vi "LED_Load_Ref-Offset.vi"(0 "Load Resource in":refnum<k15>, 1 "Max Output Resistance":string, 2 "Cluster":T1, 5 "Aperture time":dbl, 7 "Load channel name":string, 9 "DUT Current Limit":dbl, 11 "error in":errorcluster, 12 "Load voltage limit range":dbl) -> (4 "Load Resource Out":refnum<k15>, 15 "error out":errorcluster)   [LabVIEW 2021, in "start-up.lvlib"]
uses:
  start-up.lvlib
  <instrlib>/niDCPower/nidcpower.llb/niDCPower Configure Digital Edge Source Trigger With Channels.vi
  <instrlib>/niDCPower/nidcpower.llb/niDCPower Configure Digital Edge Measure Trigger With Channels.vi
  Measurement Results.ctl
  Controls/LEDStartup_Data.ctl
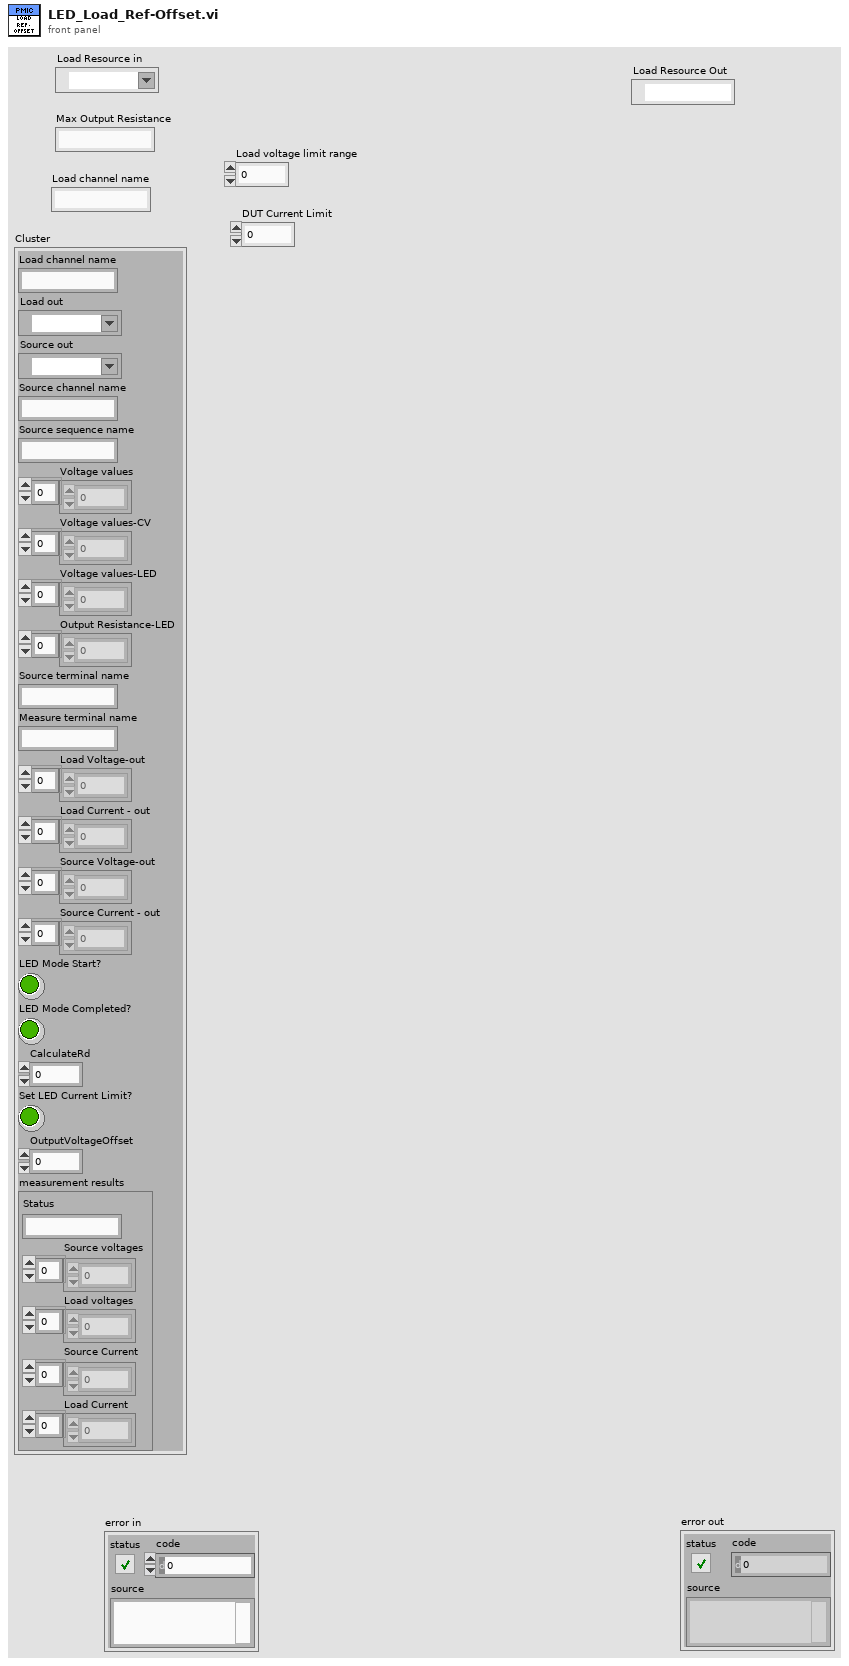
[diagram p1: front panel]
types:
  T1 = typedef "start-up.lvlib/LEDStartup_Data.ctl" = cluster{"Load channel name":string, "Load out":refnum<k15>, "Source out":refnum<k15>, "Source channel name":string, "Source sequence name":string, "Voltage values":dbl[], "Voltage values-CV":dbl[], "Voltage values-LED":dbl[], "Output Resistance-LED":dbl[], "Source terminal name":string, "Measure terminal name":string, "Load Voltage-out":dbl[], "Load Current - out":dbl[], "Source Voltage-out":dbl[], "Source Current - out":dbl[], "LED Mode Start?":bool, "LED Mode Completed?":bool, "CalculateRd":dbl, "Set LED Current Limit?":bool, "OutputVoltageOffset":dbl, "measurement results":T2}
  T2 = typedef "start-up.lvlib/Measurement Results.ctl" = cluster{"Status":string, "Source voltages":dbl[], "Load voltages":dbl[], "Source Current":dbl[], "Load Current":dbl[]}
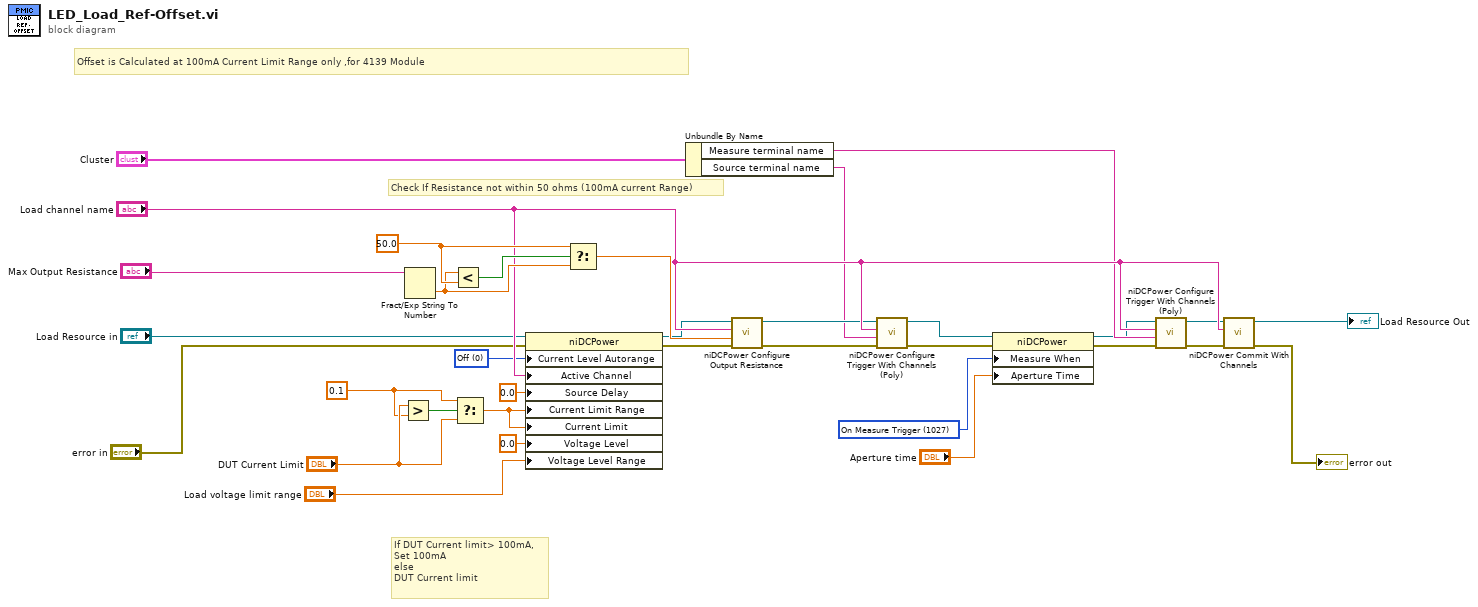
[diagram p0: block diagram]
diagram:
  w4 = 0 items=["Off", "On"] ("Source:DC Current:Current Level Autorange")
  w33 = 50.0 ("t")
  w27 = 0.1 ("y")
  w16 = 1027 items=["Automatically after Source Complete"=1025, "On Demand"=1026, "On Measure Trigger"=1027] ("Measurement:Advanced:Measure When")
  # "Offset is Calculated at 100mA Current Limit Range only ,for 4139 Module"
  # "Check If Resistance not within 50 ohms (100mA current Range)"
  # "If DUT Current limit> 100mA,\nSet 100mA\nelse\nDUT Current limit"
  n1 = Greater?(x="DUT Current Limit", y=w27) -> (0:w26:bool)
  n2 = Fract/Exp String To Number(string="Max Output Resistance") -> (number=w31:dbl)  [unwired: 3 in, 1 out]
  n3 = Less?(x=w31, y=w33) -> (x < y?=w30:bool)
  n4 = Select(t=w27, s=w26, f="DUT Current Limit") -> (s? t:f=w29:dbl)
  n5 = property class="niDCPower"(reference="Load Resource in", error in="error in", "Current Level Autorange"=w4, "Active Channel"="Load channel name", "Source Delay"=0.0 ("Source:Advanced:Source Delay"), "Current Limit Range"=w29, "Current Limit"=w29, "Voltage Level"=0.0 ("Source:DC Voltage:Voltage Level"), "Voltage Level Range"="Load voltage limit range") -> (reference out=w8:refnum<k15>, error out=w9:errorcluster)
  n6 = Select(t=w33, s=w30, f=w31) -> (s? t:f=w32:dbl)
  n7 = Unbundle By Name("Cluster") -> ("Measure terminal name"=w21:string, "Source terminal name"=w1:string)
  n8 = call <instrlib>:"niDCPower Configure Output Resistance.vi"("error in (no error)"=w9, "resistance"=w32, "channel name"="Load channel name", "instrument handle"=w8) -> ("error out"=w17:errorcluster, "instrument handle out"=w18:refnum<k15>)  [unwired: 6 in]
  n9 = call-poly <instrlib>:"niDCPower Configure Trigger With Channels (Poly).vi"("error in (no error)"=w17, "input terminal"=w1, "channel name"="Load channel name", "instrument handle"=w18) -> ("error out"=w15:errorcluster, "instrument handle out"=w10:refnum<k15>)  [unwired: 6 in]
  n10 = property class="niDCPower"(reference=w10, error in=w15, "Measure When"=w16, "Aperture Time"="Aperture time") -> (reference out=w13:refnum<k15>, error out=w14:errorcluster)
  n11 = call-poly <instrlib>:"niDCPower Configure Trigger With Channels (Poly).vi"("error in (no error)"=w14, "input terminal"=w21, "channel name"="Load channel name", "instrument handle"=w13) -> ("error out"=w12:errorcluster, "instrument handle out"=w11:refnum<k15>)  [unwired: 6 in]
  n12 = call <instrlib>:"niDCPower Commit With Channels.vi"("error in (no error)"=w12, "channel name"="Load channel name", "instrument handle"=w11) -> ("error out"=→"error out":errorcluster, "instrument handle out"=→"Load Resource Out":refnum<k15>)  [unwired: 7 in]
